vi "AIT 1553 - ReadWrite Channels.vi"(5 "Bus Section":T3, 6 "Iteration":i32, 7 "Mode":T11, 8 "error in (no error)":errorcluster, 9 "Bus Config Info":T1, 10 "FIFOs In":T12, 11 "Channels In":T4[](array[typedef]) {"Message Settings"."Driver Data"."First Word" min=8 max=31; "Message Settings"."Driver Data"."Num Bits" min=1 max=32; "Message Settings"."Driver Data"."Start Bit" min=8 max=31; "Message Settings"."Block Data Refs"."Data Reference" format="%.0x"}) -> (0 "error out":errorcluster, 2 "FIFOs Out":T12, 3 "Channels Out":T4[](array[typedef]) {"Message Settings"."Driver Data"."First Word" min=8 max=31; "Message Settings"."Driver Data"."Num Bits" min=1 max=32; "Message Settings"."Driver Data"."Start Bit" min=8 max=31; "Message Settings"."Block Data Refs"."Data Reference" format="%.0x"})   [LabVIEW 2013, in "AIT 1553 Custom Device.lvlib"]
uses:
  AIT 1553 Custom Device.lvlib
  RT Controls/FIFO.ctl
  RT Controls/ReadWrite Selector.ctl
  RT Controls/AIT 1553 - RT HW Channel.ctl
  RT Controls/AIT 1553 - Bus Section.ctl
  RT Controls/AIT 1553 - RT Message Settings.ctl
  <vilib>/NI Veristand/Custom Device API/Block Data Reference.ctl
  <vilib>/NI Veristand/Custom Device API/Data Reference.ctl
  RT Controls/AIT 1553 - Driver Data.ctl
  Controls and Global/Start Bit.ctl
  Controls and Global/Number of Bits.ctl
  RT Controls/AIT 1553 - Board Config Info.ctl
  RT Controls/AIT 1553 - Hardware Type.ctl
  <userlib>/MIL-STD-1553/vi/IBusControllerTransfer/Owl1553_IBusControllerTransfer_getLastStatusWord.vi
  <userlib>/MIL-STD-1553/vi/IBusControllerTransfer/Owl1553_IBusControllerTransfer_getErrorType.vi
  <instrlib>/AIT 1553/Public/AIT 1553 BC/Transfer/Data/AIT 1553 Read BC Xfer Message.vi
  <userlib>/MIL-STD-1553/vi/IRemoteTerminalTransfer/Owl1553_IRemoteTerminalTransfer_getLastStatusWord.vi
  <userlib>/MIL-STD-1553/vi/IRemoteTerminalTransfer/Owl1553_IRemoteTerminalTransfer_getErrorType.vi
  <instrlib>/AIT 1553/Public/AIT 1553 RT/Transfer/Data/AIT 1553 Read RT Xfer Buffer.vi
  <vilib>/NI Veristand/Custom Device Tools/Custom Device Utility Library/Custom Device Utility Library.lvlib
  <vilib>/NI Veristand/Custom Device Tools/Custom Device Utility Library/RT Debug String Color Spec.ctl
  <vilib>/NI Veristand/Custom Device API/Custom Device API.lvlib
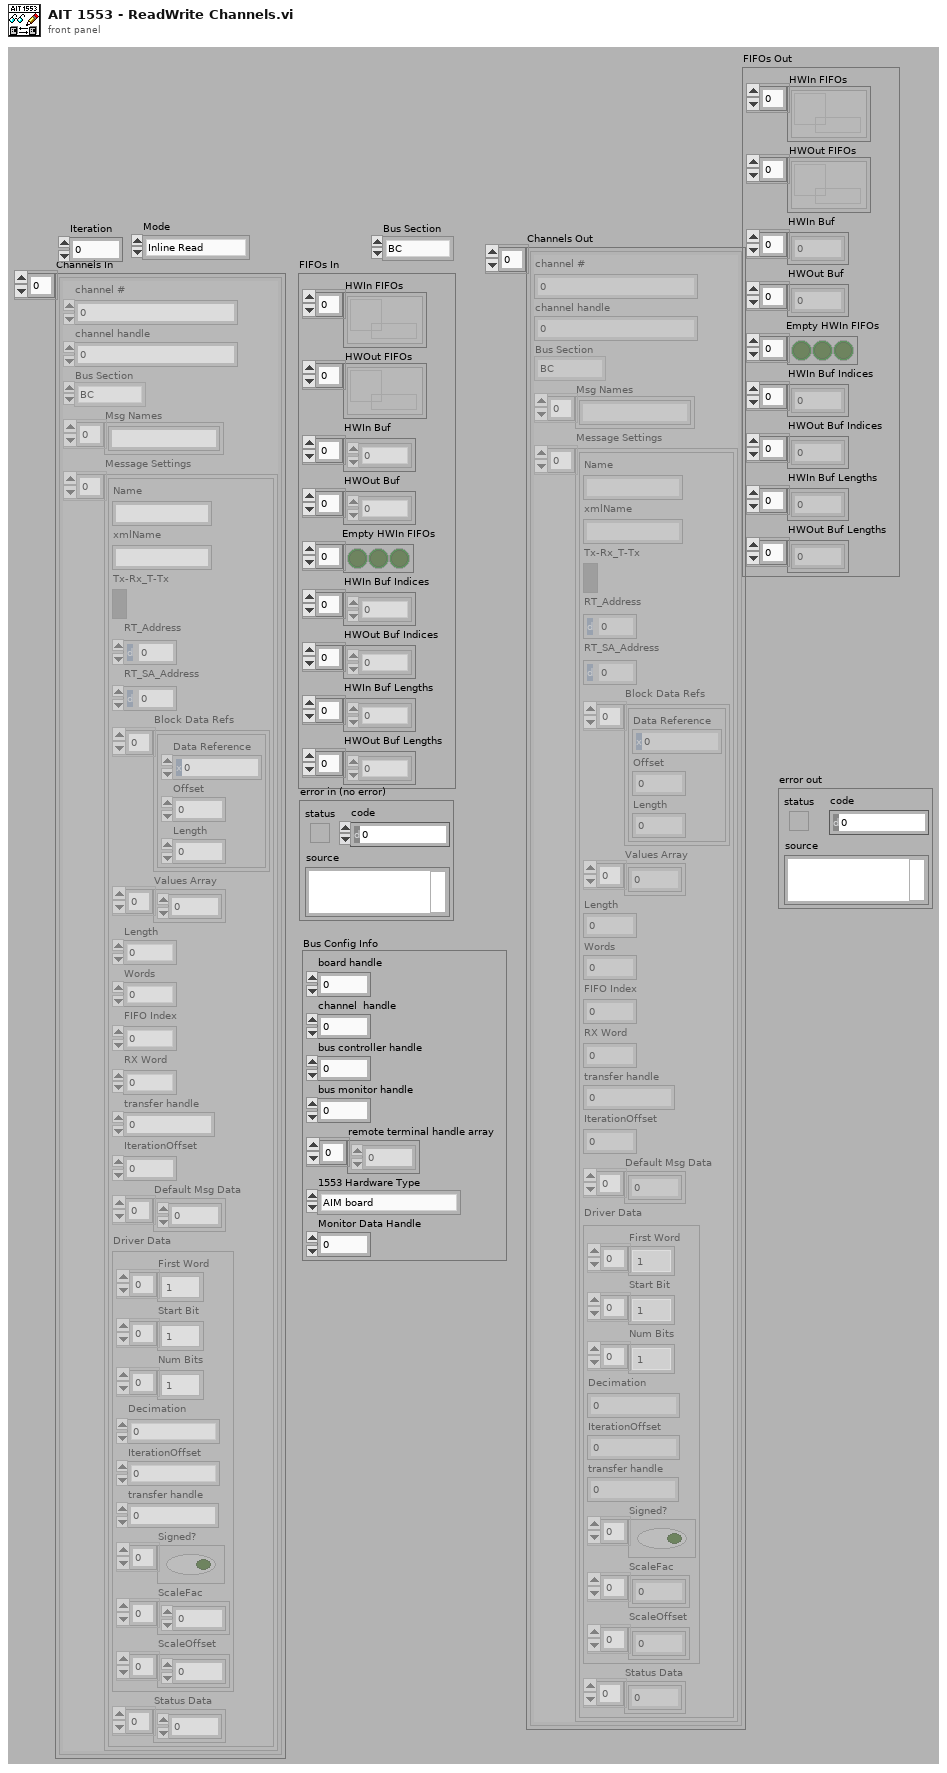
[diagram p1: front panel]
types:
  T1 = typedef "AIT 1553 Custom Device.lvlib/AIT 1553 - Board Config Info.ctl" = cluster{"board handle":u32, "channel  handle":u32, "bus controller handle":u32, "bus monitor handle":u32, "remote terminal handle array":u32[], "1553 Hardware Type":T2, "Monitor Data Handle":u32}
  T2 = typedef "AIT 1553 Custom Device.lvlib/AIT 1553 - Hardware Type.ctl" = enum16{"AIM board", "AIT Board"}
  T3 = typedef "AIT 1553 Custom Device.lvlib/AIT 1553 - Bus Section.ctl" = enum16{"BC", "BM", "RT"}
  T4 = typedef "AIT 1553 Custom Device.lvlib/AIT 1553 - RT HW Channel.ctl" = cluster{"channel #":u16, "channel handle":u32, "Bus Section":T3, "Msg Names":string[], "Message Settings":T5[]}
  T5 = typedef "AIT 1553 Custom Device.lvlib/AIT 1553 - RT Message Settings.ctl" = cluster{"Name":string, "xmlName":string, "Tx-Rx_T-Tx":bool, "RT_Address":u8, "RT_SA_Address":u8, "Block Data Refs":T6[], "Values Array":dbl[], "Length":i32, "Words":i32, "FIFO Index":i32, "RX Word":u32, "transfer handle":u32, "IterationOffset":i32, "Default Msg Data":u16[], "Driver Data":T8, "Status Data":u32[]}
  T6 = typedef "Custom Device API.lvlib/Block Data Reference.ctl" = cluster{"Data Reference":T7, "Offset":i32, "Length":i32}
  T7 = typedef "Custom Device API.lvlib/Data Reference.ctl" = i32
  T8 = typedef "AIT 1553 Custom Device.lvlib/AIT 1553 - Driver Data.ctl" = cluster{"First Word":T9[], "Start Bit":T9[], "Num Bits":T10[], "Decimation":i32, "IterationOffset":i32, "transfer handle":u32, "Signed?":bool[], "ScaleFac":dbl[], "ScaleOffset":dbl[]}
  T9 = typedef "AIT 1553 Custom Device.lvlib/Start Bit.ctl" = i32
  T10 = typedef "AIT 1553 Custom Device.lvlib/Number of Bits.ctl" = i32
  T11 = typedef "AIT 1553 Custom Device.lvlib/ReadWrite Selector.ctl" = enum16{"Inline Read", "Inline Write", "Async HWIn", "Async HWOut"}
  T12 = typedef "AIT 1553 Custom Device.lvlib/FIFO.ctl" = cluster{"HWIn FIFOs":refnum<k33>[], "HWOut FIFOs":refnum<k33>[], "HWIn Buf":dbl[], "HWOut Buf":dbl[], "Empty HWIn FIFOs":bool[], "HWIn Buf Indices":i32[], "HWOut Buf Indices":i32[], "HWIn Buf Lengths":i32[], "HWOut Buf Lengths":i32[]}
  T13 = typedef "AIT 1553 Custom Device.lvlib/VP_BM Message.ctl" = cluster{"Data Word array":u16[], "Error Exists":bool, "OWL1553_DATA_ERROR_NO_RESPONSE":bool, "Error Word":u32, "Status Word":u16, "Command Word":u16, "Time Tag - Seconds":u32, "microseconds":u32, "RT_Address":u8, "RT_SA_Address":u8, "Transmit":bool, "Msg Name":string}
  T14 = typedef "Custom Device Utility Library.lvlib/RT Debug String Color Spec.ctl" = u16
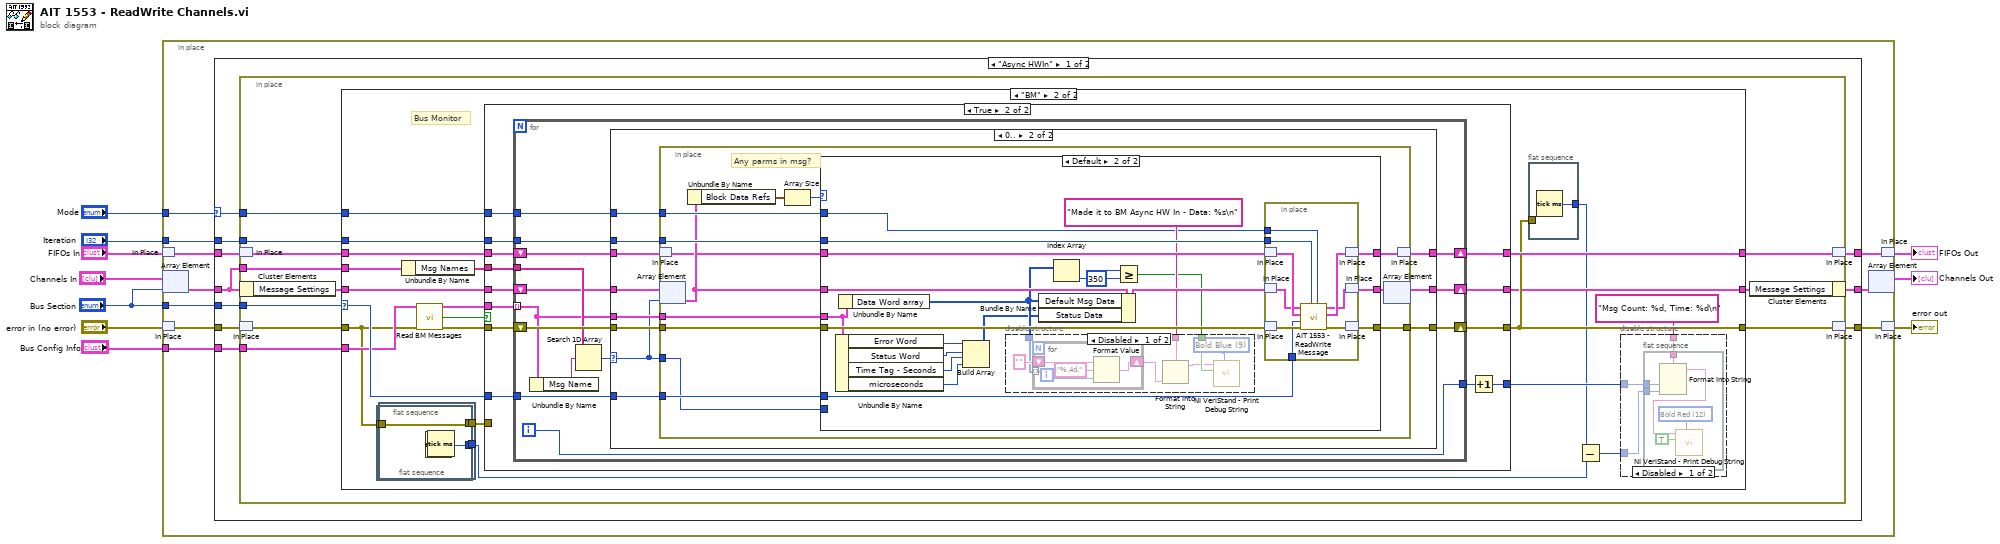
[diagram p0: block diagram]
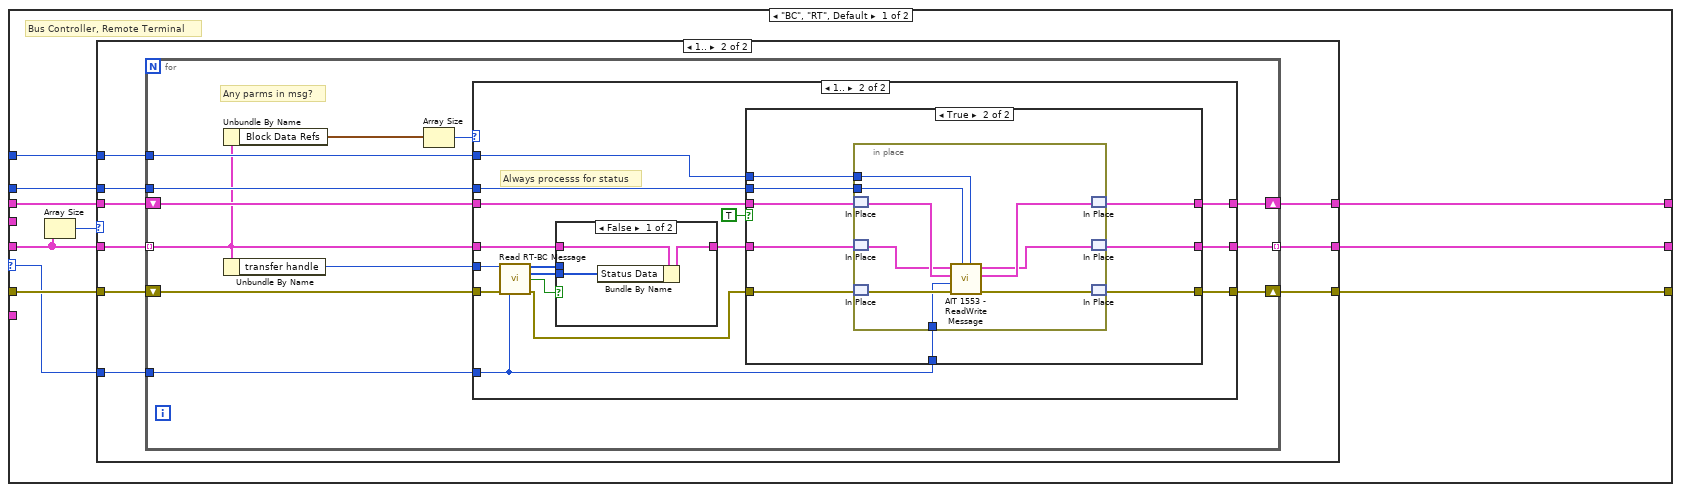
[diagram p2: hidden frame]
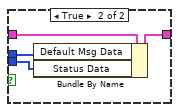
[diagram p5: hidden frame]
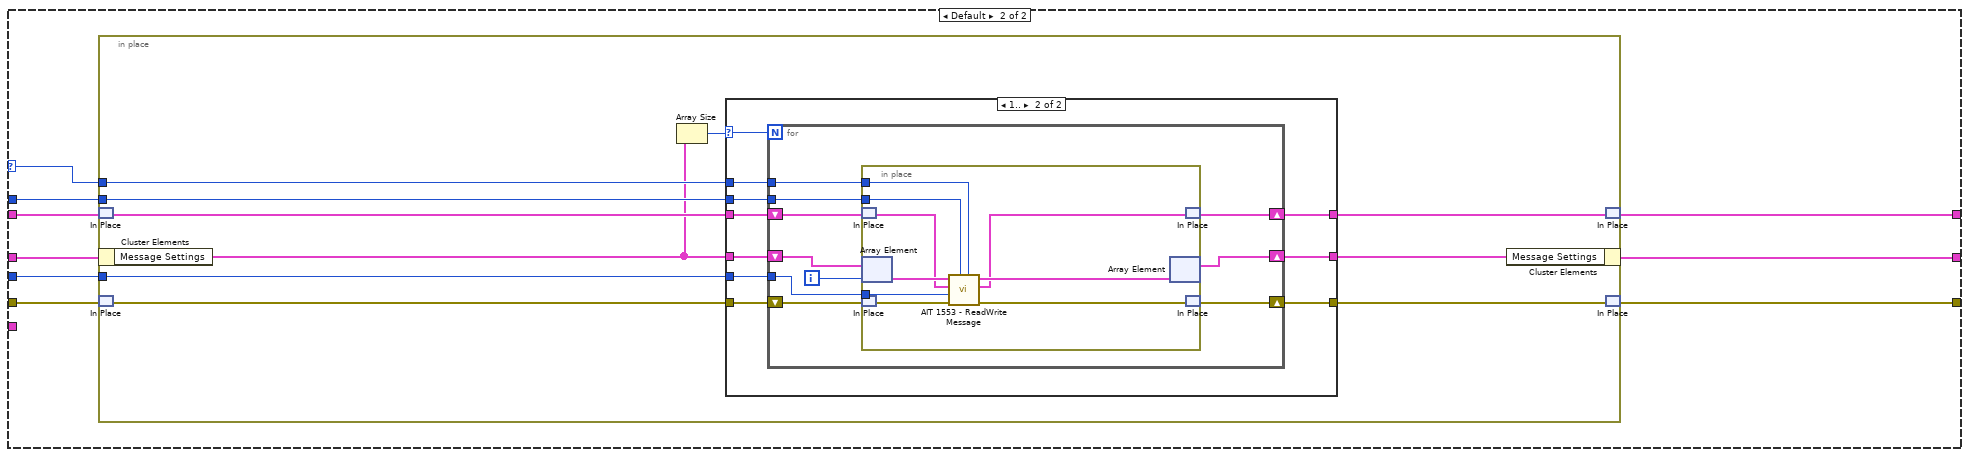
[diagram p12: hidden frame]
diagram:
  n1 = in-place {
    in-place-border: "Mode" -> [w14]
    in-place-border: "Iteration" -> [w15]
    in-place-border: "Bus Section" -> [w13]
    in-place-border: "Bus Config Info" -> [w11]
    n2 = in-place-match #1("FIFOs In") -> (w17:T12)
    n3 = in-place-array #2("Channels In", "Bus Section") -> (w12:T4)
    n4 = in-place-match #3("error in (no error)") -> (w19:errorcluster)
    n5 = case shown="\"Async HWIn\"" w14 {
      selector: w14 -> [w24 w261]
      tunnel: w12 -> [w21 w268]
      tunnel: [w30 w267] -> w20
      tunnel: w19 -> [w29 w266]
      tunnel: [w28 w265] -> w18
      tunnel: w17 -> [w27 w264]
      tunnel: [w26 w263] -> w16
      tunnel: w15 -> [w25 w262]
      tunnel: w13 -> [w23 w260]
      tunnel: w11 -> [w22 _]
      frame "Async HWIn" {
        n6 = in-place {
          in-place-border: w24 -> [w38]
          in-place-border: w25 -> [w36]
          in-place-border: w23 -> [w33]
          in-place-border: w22 -> [w32]
          in-place-border: w21 -> [w31]
          n7 = in-place-match #4(w27) -> (w35:T12)
          n8 = in-place-cluster #5(w21) -> ("Message Settings"=w41:T5[])
          n9 = in-place-match #6(w29) -> (w34:errorcluster)
          n10 = case shown="\"BM\"" w33 {
            selector: w33 -> [w44 w142]
            tunnel: w41 -> [w43 w143]
            tunnel: [w51 w125] -> w40
            tunnel: [w50 w129] -> w39
            tunnel: w38 -> [w49 w141]
            tunnel: [w48 w135] -> w37
            tunnel: w36 -> [w47 w140]
            tunnel: w35 -> [w46 w139]
            tunnel: w34 -> [w45 w131]
            tunnel: w32 -> [_ w137]
            tunnel: w31 -> [_ w133]
            frame "BC", "RT", Default {
              # "Bus Controller, Remote Terminal"
              n11 = Array Size(array=w43) -> (size(s)=w42:i32)
              n12 = case shown="1.." w42 {
                tunnel: w43 -> [w53 w63]
                tunnel: [w53 w62] -> w51
                tunnel: [w52 w61] -> w50
                tunnel: w49 -> [_ w60]
                tunnel: [w54 w59] -> w48
                tunnel: w47 -> [_ w58]
                tunnel: w46 -> [w54 w57]
                tunnel: w45 -> [w52 w56]
                tunnel: w44 -> [_ w55]
                frame 0, Default {
                }
                frame 1.. {
                  n13 = for {
                    tunnel: w63 -> [w67] mode=indexing
                    tunnel: [w65] -> w62 mode=indexing
                    tunnel: w60 -> [w74]
                    tunnel: w58 -> [w73]
                    shift-right: [w66] -> w59
                    shift-left: w57 -> [w72]
                    shift-right: [w75] -> w61
                    shift-left: w56 -> [w68]
                    tunnel: w55 -> [w64]
                    # "Any parms in msg?"
                    n14 = Unbundle By Name(w67) -> ("Block Data Refs"=w71:T6[])
                    n15 = Unbundle By Name(w67) -> ("transfer handle"=w69:u32)
                    n16 = Array Size(array=w71) -> (size(s)=w70:i32)
                    n17 = case shown="1.." w70 {
                      tunnel: w67 -> [w77 w88]
                      tunnel: [w77 w94] -> w65
                      tunnel: [w76 w93] -> w75
                      tunnel: w74 -> [_ w92]
                      tunnel: [w78 w91] -> w66
                      tunnel: w73 -> [_ w90]
                      tunnel: w72 -> [w78 w89]
                      tunnel: w69 -> [_ w87]
                      tunnel: w68 -> [w76 w86]
                      tunnel: w64 -> [_ w84]
                      frame 0, Default {
                      }
                      frame 1.. {
                        # "Always processs for status"
                        n18 = call "Read RT-BC Message.vi"("transfer handle"=w87, "error in (no error)"=w86, "Bus Section"=w84) -> ("data buffer out"=w82:u16[], "status data out"=w81:u32[], "Data Available"=w83:bool, "error out"=w80:errorcluster)  [unwired: 9 in]
                        n19 = case shown="False" w83 {
                          tunnel: w88 -> [w97 w101]
                          tunnel: [w96 w100] -> w85
                          tunnel: w82 -> [_ w99]
                          tunnel: w81 -> [w95 w98]
                          frame False {
                            n20 = Bundle By Name(cluster=w97, "Status Data"=w95) -> (w96:T5)
                          }
                          frame True {
                            n21 = Bundle By Name(cluster=w101, "Default Msg Data"=w99, "Status Data"=w98) -> (w100:T5)
                          }
                        }
                        n22 = case shown="True" TRUE {
                          tunnel: [w103 w113] -> w94
                          tunnel: [w102 w112] -> w93
                          tunnel: w92 -> [_ w111]
                          tunnel: [w104 w110] -> w91
                          tunnel: w90 -> [_ w109]
                          tunnel: w89 -> [w104 w108]
                          tunnel: w85 -> [w103 w107]
                          tunnel: w80 -> [w102 w106]
                          tunnel: w84 -> [_ w105]
                          frame False {
                            # "No Data Available"
                          }
                          frame True {
                            n23 = in-place {
                              in-place-border: w111 -> [w120]
                              in-place-border: w109 -> [w119]
                              in-place-border: w105 -> [w114]
                              n24 = in-place-match #7(w108) -> (w118:T12)
                              n25 = in-place-match #8(w107) -> (w116:T5)
                              n26 = in-place-match #9(w106) -> (w122:errorcluster)
                              n27 = call "AIT 1553 - ReadWrite Message.vi"("Mode"=w120, "Iteration"=w119, "error in (no error)"=w122, "Bus Section"=w114, "FIFOs In"=w118, "Message In"=w116) -> ("error out"=w121:errorcluster, "FIFOs Out"=w117:T12, "Message Out"=w115:T5)  [unwired: 3 in]
                              n28 = in-place-match #7(w117) -> (w110:T12)
                              n29 = in-place-match #8(w115) -> (w113:T5)
                              n30 = in-place-match #9(w121) -> (w112:errorcluster)
                            }
                          }
                        }
                      }
                    }
                  }
                }
              }
            }
            frame "BM" {
              # "Bus Monitor"
              n31 = flat-sequence {
                tunnel: [w156] -> w128
                tunnel: w131 -> [w155]
                tunnel: [w154] -> w130
                frame #0 {
                  n32 = flat-sequence {
                    tunnel: [w158] -> _
                    tunnel: w155 -> [w157]
                    tunnel: [w157] -> w154
                    frame #0 {
                      n33 = Tick Count (ms)() -> (millisecond timer value=w158:u32)
                    }
                  }
                  n34 = Tick Count (ms)() -> (millisecond timer value=w156:u32)
                }
              }
              n35 = Unbundle By Name(w133) -> ("Msg Names"=w132:string[])
              n36 = call "Read BM Messages.vi"("Bus Config Info"=w137, "error in (no error)"=w131) -> ("VP BM Messages Read"=w134:T13[], "Data Available"=w136:bool, "error out"=w138:errorcluster)  [unwired: 11 in]
              n37 = case shown="True" w136 {
                tunnel: w143 -> [w160 w174]
                tunnel: w142 -> [_ w173]
                tunnel: w141 -> [_ w172]
                tunnel: w140 -> [_ w171]
                tunnel: w139 -> [w161 w170]
                tunnel: [w160 w168] -> w125
                tunnel: [w159 w167] -> w129
                tunnel: w138 -> [w159 w166]
                tunnel: [w161 w169] -> w135
                tunnel: w134 -> [_ w165]
                tunnel: w132 -> [_ w164]
                tunnel: w130 -> [_ _]
                tunnel: [_ w162] -> w124
                frame False {
                  # "No Bus Monitor Data"
                }
                frame True {
                  n38 = for {
                    tunnel: w172 -> [w187]
                    tunnel: w171 -> [w186]
                    shift-right: [w183] -> w169
                    shift-left: w170 -> [w185]
                    shift-right: [w188] -> w167
                    shift-left: w166 -> [w184]
                    tunnel: w173 -> [w182]
                    tunnel: w165 -> [w176] mode=indexing
                    tunnel: w164 -> [w181]
                    shift-right: [w177] -> w168
                    shift-left: w174 -> [w178]
                    tunnel: [w175] -> w163
                    i -> [w175]
                    n39 = Unbundle By Name(w176) -> ("Msg Name"=w180:string)
                    n40 = Search 1D Array(1D array=w181, element=w180) -> (index of element=w179:i32)  [unwired: 1 in]
                    n41 = case shown="0.." w179 {
                      selector: w179 -> [_ w195]
                      tunnel: [w189 w202] -> w188
                      tunnel: w187 -> [_ w201]
                      tunnel: w186 -> [_ w200]
                      tunnel: w185 -> [w190 w193]
                      tunnel: w184 -> [w189 w199]
                      tunnel: [w190 w192] -> w183
                      tunnel: [w191 w194] -> w177
                      tunnel: w182 -> [_ w198]
                      tunnel: w178 -> [w191 w196]
                      tunnel: w176 -> [_ w197]
                      frame Default {
                        # "Msg not found"
                      }
                      frame 0.. {
                        n42 = in-place {
                          in-place-border: [w215] -> w202
                          in-place-border: w201 -> [w214]
                          in-place-border: w200 -> [w213]
                          in-place-border: w199 -> [w210]
                          in-place-border: w198 -> [w209]
                          in-place-border: w197 -> [w208]
                          in-place-border: w195 -> [w207]
                          # "Any parms in msg?"
                          n43 = in-place-match #10(w193) -> (w204:T12)
                          n44 = in-place-array #11(w196, w195) -> (w206:T5)
                          n45 = Unbundle By Name(w206) -> ("Block Data Refs"=w212:T6[])
                          n46 = Array Size(array=w212) -> (size(s)=w211:i32)
                          n47 = case shown="Default" w211 {
                            tunnel: w206 -> [w216 w235]
                            tunnel: [w216 w229] -> w205
                            tunnel: [w217 w239] -> w215
                            tunnel: w214 -> [_ w230]
                            tunnel: [w218 w238] -> w203
                            tunnel: w213 -> [_ w237]
                            tunnel: w204 -> [w218 w236]
                            tunnel: w210 -> [w217 w232]
                            tunnel: w209 -> [_ w233]
                            tunnel: w208 -> [_ w224]
                            tunnel: w207 -> [_ _]
                            frame ..0 {
                            }
                            frame Default {
                              n48 = Unbundle By Name(w224) -> ("Error Word"=w223:u32, "Status Word"=w222:u16, "Time Tag - Seconds"=w221:u32, "microseconds"=w220:u32)
                              n49 = Unbundle By Name(w224) -> ("Data Word array"=w228:u16[])
                              n50 = Build Array(w223, w222, w221, w220) -> (w219:u32[])
                              n51 = Bundle By Name(cluster=w235, "Default Msg Data"=w228, "Status Data"=w219) -> (w234:T5)
                              n52 = Index Array(array=w228) -> (element=w227:u16)  [unwired: 1 in]
                              n53 = Greater Or Equal?(x=w227, y=u16 350) -> (x >= y?=w225:bool)
                              n54 = disable-structure shown="Disabled" {
                                disable-tunnel: "Made it to BM Async HW In - Data: %s\n" ("format string") -> [w245 _]
                                disable-tunnel: w228 -> [w243 _]
                                disable-tunnel: w225 -> [w242 _]
                                frame Disabled {
                                w240 = T14 9 items=["Plain White"=7, "Bold White"=15, "Bold Blue"=9, "Bold Green"=10, "Bold Red"=12] ("Attribute")
                                n55 = for {
                                tunnel: w243 -> [w247] mode=indexing
                                shift-right: [w248] -> w244
                                shift-left: "" ("format string") -> [w249]
                                n56 = Format Value(string ("")=w249, format string="%.4d,", value (0)=w247) -> (output string=w248:string)
                                }
                                n57 = Format Into String(format string=w245, w244) -> (resulting string=w241:string)  [unwired: 2 in, 1 out]
                                n58 = call <vilib>:"NI VeriStand - Print Debug String.vi"("Attribute"=w240, "Add to log file? (T)"=w242, "Message"=w241) -> ()  [unwired: 8 in, 1 out]
                                }
                                frame Enabled {
                                }
                              }
                              n59 = in-place {
                                in-place-border: w230 -> [w257]
                                in-place-border: w237 -> [w256]
                                in-place-border: w233 -> [w251]
                                n60 = in-place-match #12(w236) -> (w255:T12)
                                n61 = in-place-match #13(w234) -> (w253:T5)
                                n62 = in-place-match #14(w232) -> (w259:errorcluster)
                                n63 = call "AIT 1553 - ReadWrite Message.vi"("Mode"=w257, "Iteration"=w256, "error in (no error)"=w259, "Bus Section"=w251, "FIFOs In"=w255, "Message In"=w253) -> ("error out"=w258:errorcluster, "FIFOs Out"=w254:T12, "Message Out"=w252:T5)  [unwired: 3 in]
                                n64 = in-place-match #12(w254) -> (w238:T12)
                                n65 = in-place-match #13(w252) -> (w229:T5)
                                n66 = in-place-match #14(w258) -> (w239:errorcluster)
                              }
                            }
                          }
                          n67 = in-place-array #11(w205) -> (w194:T5[])  [unwired: 1 out]
                          n68 = in-place-match #10(w203) -> (w192:T12)
                        }
                      }
                    }
                  }
                  n69 = Increment(x=w163) -> (x+1=w162:i32)
                }
              }
              n70 = flat-sequence {
                tunnel: [w153] -> w123
                tunnel: w129 -> [_]
                frame #0 {
                  n71 = Tick Count (ms)() -> (millisecond timer value=w153:u32)
                }
              }
              n72 = Subtract(x=w123, y=w128) -> (x-y=w126:u32)
              n73 = disable-structure shown="Disabled" {
                disable-tunnel: "Msg Count: %d, Time: %d\n" ("format string") -> [w146 _]
                disable-tunnel: w126 -> [w145 _]
                disable-tunnel: w124 -> [w144 _]
                frame Disabled {
                  n74 = flat-sequence {
                    tunnel: w146 -> [w152]
                    tunnel: w145 -> [w151]
                    tunnel: w144 -> [w150]
                    frame #0 {
                      w149 = T14 12 items=["Plain White"=7, "Bold White"=15, "Bold Blue"=9, "Bold Green"=10, "Bold Red"=12] ("Attribute")
                      n75 = Format Into String(format string=w152, w150, w151) -> (resulting string=w147:string)  [unwired: 2 in, 1 out]
                      n76 = call <vilib>:"NI VeriStand - Print Debug String.vi"("Attribute"=w149, "Add to log file? (T)"=TRUE, "Message"=w147) -> ()  [unwired: 8 in, 1 out]
                    }
                  }
                }
                frame Enabled {
                }
              }
            }
          }
          n77 = in-place-cluster #5("Message Settings"=w40) -> (w30:T4)
          n78 = in-place-match #4(w37) -> (w26:T12)
          n79 = in-place-match #6(w39) -> (w28:errorcluster)
        }
      }
      frame Default {
        n80 = in-place {
          in-place-border: w261 -> [w276]
          in-place-border: w262 -> [w274]
          in-place-border: w260 -> [w270]
          n81 = in-place-match #15(w264) -> (w273:T12)
          n82 = in-place-cluster #16(w268) -> ("Message Settings"=w271:T5[])
          n83 = in-place-match #17(w266) -> (w272:errorcluster)
          n84 = Array Size(array=w271) -> (size(s)=w269:i32)
          n85 = case shown="1.." w269 {
            selector: w269 -> [_ w282]
            tunnel: [w280 w291] -> w278
            tunnel: [w279 w290] -> w277
            tunnel: w276 -> [_ w289]
            tunnel: [w281 w288] -> w275
            tunnel: w274 -> [_ w287]
            tunnel: w273 -> [w281 w286]
            tunnel: w272 -> [w279 w285]
            tunnel: w271 -> [w280 w284]
            tunnel: w270 -> [_ w283]
            frame 0, Default {
            }
            frame 1.. {
              n86 = for {
                N: w282 -> [_]
                shift-right: [w297] -> w290
                shift-left: w285 -> [w298]
                tunnel: w289 -> [w296]
                tunnel: w287 -> [w293]
                shift-right: [w294] -> w288
                shift-left: w286 -> [w295]
                shift-right: [w299] -> w291
                shift-left: w284 -> [w301]
                tunnel: w283 -> [w292]
                i -> [w300]
                n87 = in-place {
                  in-place-border: w296 -> [w307]
                  in-place-border: w293 -> [w308]
                  in-place-border: w292 -> [w302]
                  n88 = in-place-match #18(w295) -> (w303:T12)
                  n89 = in-place-array #19(w301, w300) -> (w304:T5)
                  n90 = in-place-match #20(w298) -> (w305:errorcluster)
                  n91 = call "AIT 1553 - ReadWrite Message.vi"("Mode"=w307, "Iteration"=w308, "error in (no error)"=w305, "Bus Section"=w302, "FIFOs In"=w303, "Message In"=w304) -> ("error out"=w310:errorcluster, "FIFOs Out"=w306:T12, "Message Out"=w309:T5)  [unwired: 3 in]
                  n92 = in-place-array #19(w309) -> (w299:T5[])  [unwired: 1 out]
                  n93 = in-place-match #18(w306) -> (w294:T12)
                  n94 = in-place-match #20(w310) -> (w297:errorcluster)
                }
              }
            }
          }
          n95 = in-place-cluster #16("Message Settings"=w278) -> (w267:T4)
          n96 = in-place-match #15(w275) -> (w263:T12)
          n97 = in-place-match #17(w277) -> (w265:errorcluster)
        }
      }
    }
    n98 = in-place-array #2(w20) -> (→"Channels Out":T4[])  [unwired: 1 out]
    n99 = in-place-match #1(w16) -> (→"FIFOs Out":T12)
    n100 = in-place-match #3(w18) -> (→"error out":errorcluster)
  }
